vi "configure_awg.vi"(0 "VISA name":refnum<visa-resource-name>="AWG5014", 1 "Ref. Amplitude":dbl=1.0, 2 "Sum Name":string="ipsum", 3 "Ref. Name":string="lorem", 5 "Frequency":dbl=40000000.0, 7 "Max sample rate":dbl=1200000000.0, 9 "Cant. Freq":dbl=5000.0, 11 "Wipe Names on execute":bool, 12 "Amp 1":dbl=1.0, 14 "Amp 2":dbl=1.0) -> ()   [LabVIEW 2018]
uses:
  <instrlib>/Tektronix AWG 5000 7000 Series/Public/Configure/Channel/Assign Output Waveform (From Waveform List).vi
  <instrlib>/Tektronix AWG 5000 7000 Series/Tektronix AWG 5000 7000 Series.lvlib
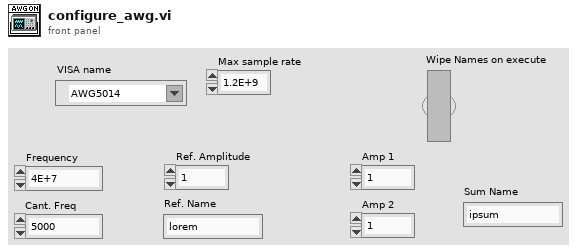
[diagram p1: front panel]
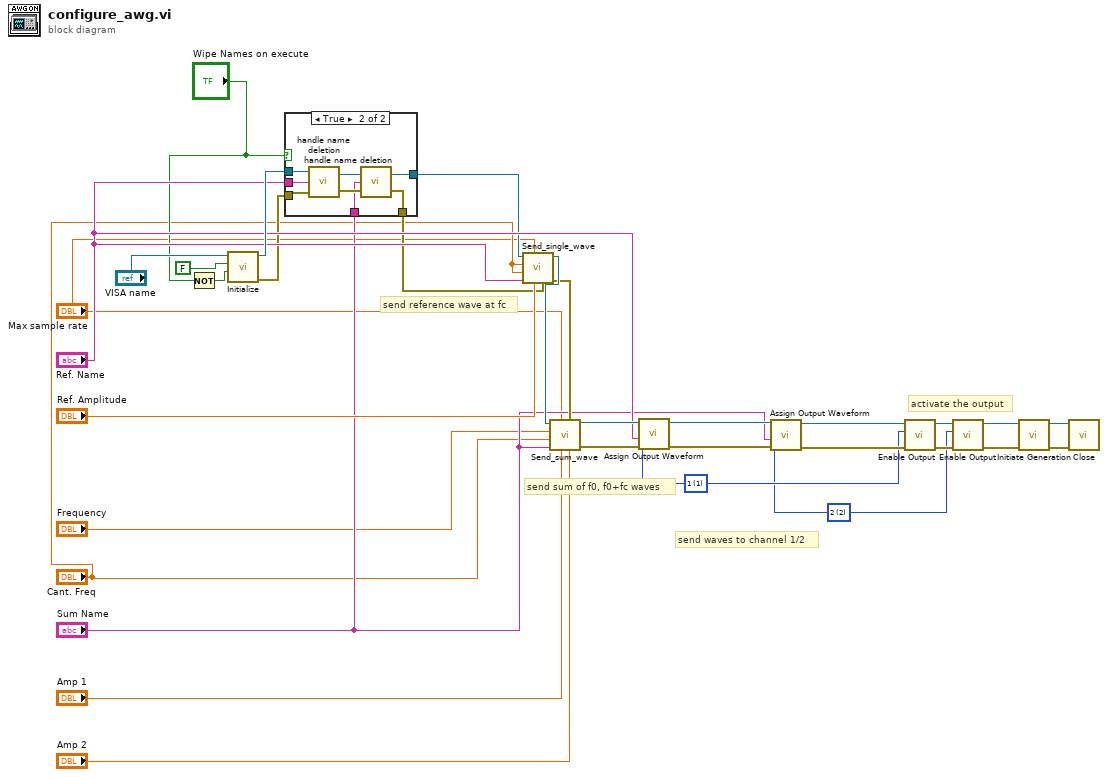
[diagram p0: block diagram]
diagram:
  w19 = u16 1 items=["1"=1, "2"=2, "3"=3, "4"=4] ("Channel Name (1)")
  w16 = u16 2 items=["1"=1, "2"=2, "3"=3, "4"=4] ("Channel Name (1)")
  # "activate the output"
  # "send waves to channel 1/2"
  # "send sum of f0, f0+fc waves"
  # "send reference wave at fc"
  n1 = Not(x="Wipe Names on execute") -> (.not. x?=w6:bool)
  n2 = call <instrlib>:"Initialize.vi"("Reset (False)"=w6, "ID Query (True)"=FALSE, "VISA resource name"="VISA name") -> ("error out"=w9:errorcluster, "VISA resource name out"=w11:refnum<visa-resource-name>)  [unwired: 7 in]
  n3 = case shown="True" "Wipe Names on execute" {
    tunnel: w11 -> [w33 w42]
    tunnel: "Ref. Name" -> [_ w41]
    tunnel: w9 -> [w34 w40]
    tunnel: [w33 w39] -> w8
    tunnel: [w34 w38] -> w7
    tunnel: "Sum Name" -> [_ w35]
    frame False {
    }
    frame True {
      n4 = call "handle name deletion.vi"("error in (no error)"=w40, "String"=w41, "VISA resource name"=w42) -> ("error out"=w36:errorcluster, "VISA resource name out"=w37:refnum<visa-resource-name>)
      n5 = call "handle name deletion.vi"("error in (no error)"=w36, "String"=w35, "VISA resource name"=w37) -> ("error out"=w38:errorcluster, "VISA resource name out"=w39:refnum<visa-resource-name>)
    }
  }
  n6 = call "Send_single_wave.vi"("error in (no error)"=w7, "Amplitude"="Ref. Amplitude", "Max sample rate"="Max sample rate", "Name"="Ref. Name", "Cant. Freq"="Cant. Freq", "Frequency"="Cant. Freq", "VISA resource name"=w8) -> ("error out"=w28:errorcluster, "VISA resource name out"=w29:refnum<visa-resource-name>)  [unwired: 3 in]
  n7 = call "Send_sum_wave.vi"("Amp 2"="Amp 2", "error in (no error)"=w28, "Amp 1"="Amp 1", "Max sample rate"="Max sample rate", "Name"="Sum Name", "Cant. Freq"="Cant. Freq", "Frequency"="Frequency", "VISA resource name"=w29) -> ("error out"=w24:errorcluster, "VISA resource name out"=w25:refnum<visa-resource-name>)  [unwired: 2 in]
  n8 = call-poly <instrlib>:"Assign Output Waveform.vi"("error in (no error)"=w24, "Waveform"="Ref. Name", "Channel Name (1)"=w19, "VISA resource name"=w25) -> ("error out"=w22:errorcluster, "VISA resource name out"=w23:refnum<visa-resource-name>)  [unwired: 6 in]
  n9 = call-poly <instrlib>:"Assign Output Waveform.vi"("error in (no error)"=w22, "Waveform"="Sum Name", "Channel Name (1)"=w16, "VISA resource name"=w23) -> ("error out"=w20:errorcluster, "VISA resource name out"=w21:refnum<visa-resource-name>)  [unwired: 6 in]
  n10 = call <instrlib>:"Enable Output.vi"("error in (no error)"=w20, "Channel Name (1)"=w19, "VISA resource name"=w21) -> ("error out"=w17:errorcluster, "VISA resource name out"=w18:refnum<visa-resource-name>)  [unwired: 7 in]
  n11 = call <instrlib>:"Enable Output.vi"("error in (no error)"=w17, "Channel Name (1)"=w16, "VISA resource name"=w18) -> ("error out"=w14:errorcluster, "VISA resource name out"=w15:refnum<visa-resource-name>)  [unwired: 7 in]
  n12 = call <instrlib>:"Initiate Generation.vi"("error in (no error)"=w14, "VISA resource name"=w15) -> ("error out"=w12:errorcluster, "VISA resource name out"=w13:refnum<visa-resource-name>)  [unwired: 8 in]
  n13 = call <instrlib>:"Close.vi"("error in (no error)"=w12, "VISA resource name"=w13) -> ()  [unwired: 9 in, 1 out]
